vi "Substitute Actor.vi"(10 "Substitute Actor in":refnum<class "Actor.lvclass">, 11 "Current Chef State":refnum<class "Chef State.lvclass">) -> (0 "error out":errorcluster, 2 "Substitute Actor out":refnum<class "Actor.lvclass">)   [LabVIEW 2021, in "Chef States.lvlib" / "Chef State.lvclass"]
doc: "(<B>Filename</B>: Actor Framework.lvlib:Actor.lvclass:Substitute Actor.vi)\n\nThis method copies information from the <b>Current Actor</b> to the <b>Substitute Actor</b>, including the to-self and the to-caller queue references. The purpose of this function is to allow an actor to define a method that replaces itself with another actor, useful for implementing a State Pattern Actor. Child classes should override this method to copy any additional fields that they need from the current to the substitute.\n\nThis method may return error code 678010: Illegal substitution. Overrides of this method may choose to return this error if the new actor is not one that is an appropriate substitute for the current actor, for whatever standards of \"appropriate\" are chosen for the current actor. If returning an error, override VIs should return the unmodified <b>Current Actor</b> as <b>Substitute Actor out</b>."
uses:
  Chef State.lvclass
  <vilib>/NI/Actors/State Actor/State Actor/State Actor.lvclass
  <vilib>/ActorFramework/Actor/Actor.lvclass
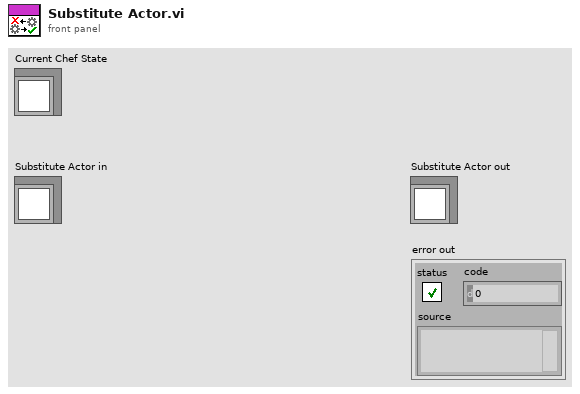
[diagram p1: front panel]
types:
  T1 = cluster{"Kitchen":refnum<class "Message Enqueuer.lvclass">}
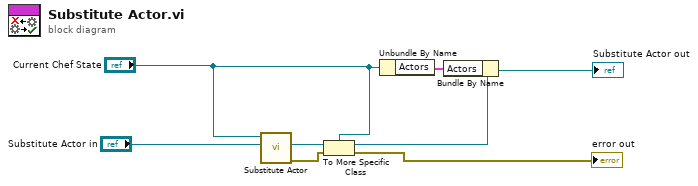
[diagram p0: block diagram]
diagram:
  n1 = call-parent "Substitute Actor.vi"("Substitute Actor in"="Substitute Actor in", "Current Actor"="Current Chef State") -> ("error out"=w4:errorcluster, "Substitute Actor out"=w8:refnum<class "Actor.lvclass">)  [unwired: 8 in]
  n2 = To More Specific Class(target class="Current Chef State", reference=w8, error in=w4) -> (specific class reference=w5:refnum<class "Chef State.lvclass">, error out=→"error out":errorcluster)
  n3 = Unbundle By Name("Current Chef State") -> ("Actors"=w1:T1)
  n4 = Bundle By Name(cluster=w5, "Actors"=w1) -> (→"Substitute Actor out":refnum<class "Chef State.lvclass">)
